vi "Calculate Messages.vi"(8 "error in (no error)":errorcluster, 11 "Tree Reference":refnum<vi>) -> (0 "error out":errorcluster, 3 "Array of Messages to be build":string[](array[string]))   [LabVIEW 2014, in "CS++MessageMakerMain.lvlib" / "CS++MessageMakerMain.lvclass"]
doc: "Helper VI to calculate which Messages should be created."
uses:
  CS++MessageMakerMain.lvclass
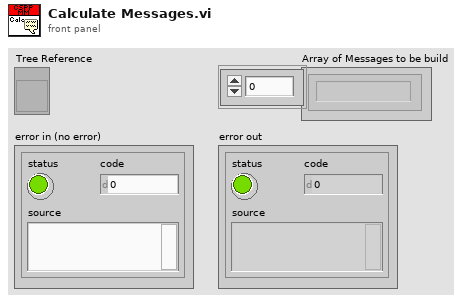
[diagram p1: front panel]
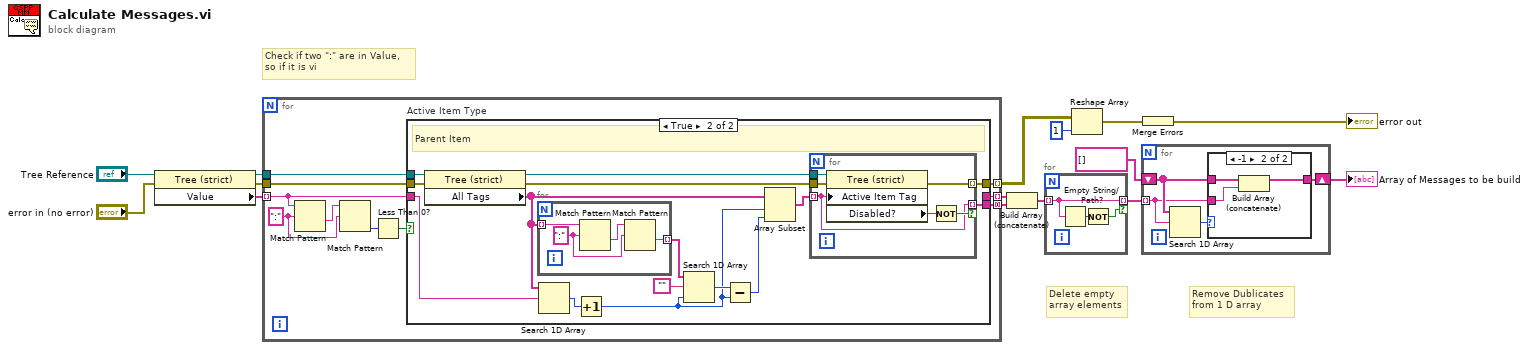
[diagram p0: block diagram]
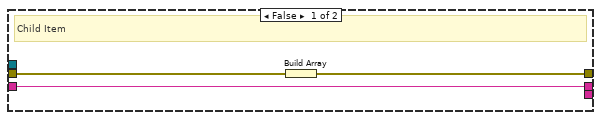
[diagram p3: hidden frame]
diagram:
  # "Remove Dublicates\nfrom 1 D array"
  # "Delete empty\narray elements"
  # "Check if two \":\" are in Value,\nso if it is vi"
  n1 = property class="Tree (strict)"(reference="Tree Reference", error in="error in (no error)") -> (reference out=w14:refnum<vi>, error out=w12:errorcluster, "Value"=w15:string[])
  n2 = for {
    tunnel: w15 -> [w20] mode=indexing
    tunnel: w14 -> [w25]
    tunnel: [w19] -> w13 mode=indexing
    tunnel: w12 -> [w18]
    tunnel: [w17] -> w11 mode=concatenating
    tunnel: [w16] -> w5 mode=indexing
    w23 = ":" ("regular expression")
    n3 = Match Pattern(string=w20, regular expression=w23) -> (after substring=w24:string)  [unwired: 1 in, 3 out]
    n4 = Match Pattern(string=w24, regular expression=w23) -> (offset past match=w22:i32)  [unwired: 1 in, 3 out]
    n5 = Less Than 0?(x=w22) -> (x < 0?=w21:bool)
    n6 = case "Active Item Type" shown="True" w21 {
      tunnel: w25 -> [_ w43]
      tunnel: w20 -> [w28 w41]
      tunnel: [w28 _] -> w19
      tunnel: w18 -> [w27 w42]
      tunnel: [_ w31] -> w17
      tunnel: [w26 w29] -> w16
      frame False {
        # "Child Item"
        n7 = Build Array(w27) -> (w26:errorcluster[])
      }
      frame True {
        # "Parent Item"
        n8 = property class="Tree (strict)"(reference=w43, error in=w42) -> (reference out=w33:refnum<vi>, error out=w32:errorcluster, "All Tags"=w37:string[])
        n9 = for {
          tunnel: w37 -> [w51] mode=indexing
          tunnel: [w50] -> w39 mode=indexing
          w52 = ":" ("regular expression")
          n10 = Match Pattern(string=w51, regular expression=w52) -> (after substring=w53:string)  [unwired: 1 in, 3 out]
          n11 = Match Pattern(string=w53, regular expression=w52) -> (after substring=w50:string)  [unwired: 1 in, 3 out]
        }
        n12 = Search 1D Array(1D array=w37, element=w41) -> (index of element=w40:i32)  [unwired: 1 in]
        n13 = Increment(x=w40) -> (x+1=w30:i32)
        n14 = Search 1D Array(1D array=w39, element="", start index (0)=w30) -> (index of element=w36:i32)
        n15 = Subtract(x=w36, y=w30) -> (x-y=w35:i32)
        n16 = Array Subset(array=w37, index=w30, length=w35) -> (w34:string[])
        n17 = for {
          tunnel: w34 -> [w45] mode=indexing
          tunnel: w33 -> [w49]
          tunnel: w32 -> [w48]
          tunnel: [w45] -> w31 mode=indexing if=w46
          tunnel: [w44] -> w29 mode=indexing
          n18 = property class="Tree (strict)"(reference=w49, error in=w48, "Active Item Tag"=w45) -> (error out=w44:errorcluster, "Disabled?"=w47:bool)  [unwired: 1 out]
          n19 = Not(x=w47) -> (.not. x?=w46:bool)
        }
      }
    }
  }
  n20 = Build Array (concatenate)(w13, w11) -> (w9:string[])
  n21 = for {
    tunnel: w9 -> [w56] mode=indexing
    tunnel: [w56] -> w8 mode=indexing if=w54
    n22 = Empty String/Path?(string/path=w56) -> (empty?=w55:bool)
    n23 = Not(x=w55) -> (.not. x?=w54:bool)
  }
  n24 = Reshape Array(w5, 1 ("dimension size")) -> (w3:errorcluster[])
  n25 = for {
    tunnel: w8 -> [w57] mode=indexing
    shift-right: [w58] -> w1
    shift-left: string[] [] -> [w59]
    n26 = Search 1D Array(1D array=w59, element=w57) -> (index of element=w60:i32)  [unwired: 1 in]
    n27 = case shown="-1" w60 {
      tunnel: w59 -> [w61 w64]
      tunnel: [w61 w63] -> w58
      tunnel: w57 -> [_ w62]
      frame 0.., Default {
      }
      frame -1 {
        n28 = Build Array (concatenate)(w64, w62) -> (w63:string[])
      }
    }
  }
  "Array of Messages to be build" <- w1
  n29 = Merge Errors(w3) -> (→"error out":errorcluster)
